vi "Test Panel Position.vi"() -> ()   [LabVIEW 2013]
uses:
  Type Defs/AD Settings.ctl
  Type Defs/Output Values.ctl
  Type Defs/Output Switches.ctl
  Type Defs/CO2 Settings.ctl
  Type Defs/Final Output for Dispaly 2.ctl
  Type Defs/Data Reading.ctl
  Type Defs/Named Final Output name list ordered.ctl
  Type Defs/All Timers.ctl
  Type Defs/Timer Control.ctl
  Altitude/Altitude.xctl
  Type Defs/Action Time.ctl
  Mode Control/Mode.xctl
  Type Defs/Current Alt Set.ctl
  Type Defs/Alt Control.ctl
  Type Defs/Alt Digit 100 New.ctl
  MSR/VertMode/VertMode.xctl
  Type Defs/Named Final Output name list with 02.ctl
  Type Defs/Alt Display Large.ctl
  <vilib>/Utility/miscctls.llb/LVPositionTypeDef.ctl
  <vilib>/Utility/miscctls.llb/LVRectTypeDef.ctl
  <vilib>/Utility/miscctls.llb/LVPointTypeDef.ctl
panel:
  out "Position":T1
  out "read string":string="Ver. 0.9, May 29 2013, 00:37:20\r\n"
  in  "Main Tabs":T2(tab)=enum."CO2 Settings"
  in  "Other Outputs":cluster{"Alarm":bool, "Heater":bool}
  out "CO2 ppm":u32(slide)=493 scale=0.0..10000.0
  out "Alt Dif":dbl(slide)=1604.2180978990014 scale=-1000.0..1000.0 scale format="%.1f"
  out "AD Output":T3
  out "AD State":T3
  out "Data Read":T4={"Date"="06/07/13", "Time"="14:45:26", "CO2- ppm"=493, "Last Ctrl Word"=12582912, "O2-1 ppm"=209797, "O2-2 ppm"=209799, "Temp MB"=26.17, "Temp Sensor Module"=27.17, "Press mB"=833.31} {"Last Ctrl Word" format="%.0x"}
  out "Force Output":T3
  out "Final Output":T3
  out "Force State":T3
  in  "CO2 Settings":T5={"Run C1"={"A-1,  1"=inf, "A-3,  2"=inf, "A-4, 3"=9600.0, "A-5, 4"=8800.0, "ABCD-7, 5"=9800.0, "A-8, 6"=9800.0, "B-1,  7"=3400.0, "B-3, 8"=3400.0, "B-4,  9"=9600.0, "B-5, 10"=8800.0, "B-8, 11"=9800.0, "C-1, 12"=1800.0, "C-3, 13"=1800.0, "C-4, 14"=9600.0, "C-5,  15"=8800.0, "C-8, 16"=9800.0, "D-1, 17"=inf, "D-3, 18"=3400.0, "D-4,  19"=1800.0, "D-5,  20"=9800.0, "D-8,  21"=9800.0}, "Run C2"={"A-1,  1"=inf, "A-3,  2"=inf, "A-4, 3"=9500.0, "A-5, 4"=8600.0, "ABCD-7, 5"=9700.0, "A-8, 6"=9700.0, "B-1,  7"=3000.0, "B-3, 8"=3000.0, "B-4,  9"=9500.0, "B-5, 10"=8600.0, "B-8, 11"=9700.0, "C-1, 12"=1400.0, "C-3, 13"=1400.0, "C-4, 14"=9500.0, "C-5,  15"=8600.0, "C-8, 16"=9700.0, "D-1, 17"=inf, "D-3, 18"=3000.0, "D-4,  19"=1400.0, "D-5,  20"=9700.0, "D-8,  21"=9700.0}, "Hold C3"={"A-1,  1"=1800.0, "A-3,  2"=1800.0, "A-4, 3"=9000.0, "A-5, 4"=8800.0, "ABCD-7, 5"=9800.0, "A-8, 6"=9800.0, "B-1,  7"=3400.0, "B-3, 8"=3400.0, "B-4,  9"=9000.0, "B-5, 10"=8800.0, "B-8, 11"=9800.0, "C-1, 12"=1800.0, "C-3, 13"=1800.0, "C-4, 14"=9000.0, "C-5,  15"=8800.0, "C-8, 16"=9800.0, "D-1, 17"=1800.0, "D-3, 18"=3400.0, "D-4,  19"=1800.0, "D-5,  20"=9800.0, "D-8,  21"=9800.0}, "Hold C4"={"A-1,  1"=1400.0, "A-3,  2"=1400.0, "A-4, 3"=8800.0, "A-5, 4"=8600.0, "ABCD-7, 5"=9700.0, "A-8, 6"=9700.0, "B-1,  7"=3000.0, "B-3, 8"=3000.0, "B-4,  9"=8800.0, "B-5, 10"=8600.0, "B-8, 11"=9700.0, "C-1, 12"=1400.0, "C-3, 13"=1400.0, "C-4, 14"=8800.0, "C-5,  15"=8600.0, "C-8, 16"=9700.0, "D-1, 17"=1400.0, "D-3, 18"=3000.0, "D-4,  19"=1400.0, "D-5,  20"=9700.0, "D-8,  21"=9700.0}, "High CO2 Forces"={"A-1, 1"=TRUE, "A-3, 2"=TRUE, "A-4, 3"=FALSE, "A-5, 4"=TRUE, "ABCD-7, 5"=FALSE, "A-8, 6"=TRUE, "B-1,  7"=TRUE, "B-3, 8"=TRUE, "B-4, 9"=FALSE, "B-5, 10"=TRUE, "B-8,  11"=TRUE, "C-1, 12"=TRUE, "C-3, 13"=TRUE, "C-4,  14"=FALSE, "C-5,  15"=TRUE, "C-8, 16"=TRUE, "D-1, 17"=TRUE, "D-3, 18"=TRUE, "D-4, 19"=TRUE, "D-5,  20"=TRUE, "D-8,  21"=TRUE}}
  in  "AD Settings":T8={"Set Point Force"={"A-1,  1"=inf, "A-3,  2"=inf, "A-4, 3"=inf, "A-5, 4"=5790.0, "ABCD-7, 5"=inf, "A-8, 6"=inf, "B-1,  7"=5790.0, "B-3, 8"=5790.0, "B-4,  9"=inf, "B-5, 10"=5790.0, "B-8, 11"=inf, "C-1, 12"=inf, "C-3, 13"=inf, "C-4, 14"=inf, "C-5,  15"=5790.0, "C-8, 16"=inf, "D-1, 17"=inf, "D-3, 18"=inf, "D-4,  19"=inf, "D-5,  20"=inf, "D-8,  21"=inf}, "Run A1"={"A-1,  1"=inf, "A-3,  2"=inf, "A-4, 3"=3.0, "A-5, 4"=inf, "ABCD-7, 5"=67.0, "A-8, 6"=630.0, "B-1,  7"=-30.0, "B-3, 8"=-30.0, "B-4,  9"=3.0, "B-5, 10"=inf, "B-8, 11"=630.0, "C-1, 12"=-60.0, "C-3, 13"=-60.0, "C-4, 14"=3.0, "C-5,  15"=inf, "C-8, 16"=630.0, "D-1, 17"=inf, "D-3, 18"=-30.0, "D-4,  19"=-60.0, "D-5,  20"=630.0, "D-8,  21"=930.0}, "Run A2"={"A-1,  1"=inf, "A-3,  2"=inf, "A-4, 3"=-3.0, "A-5, 4"=inf, "ABCD-7, 5"=60.0, "A-8, 6"=610.0, "B-1,  7"=-100.0, "B-3, 8"=-100.0, "B-4,  9"=-3.0, "B-5, 10"=inf, "B-8, 11"=610.0, "C-1, 12"=-120.0, "C-3, 13"=-120.0, "C-4, 14"=-3.0, "C-5,  15"=inf, "C-8, 16"=610.0, "D-1, 17"=inf, "D-3, 18"=-100.0, "D-4,  19"=-120.0, "D-5,  20"=610.0, "D-8,  21"=910.0}, "Hold A3"={"A-1,  1"=0.0, "A-3,  2"=0.0, "A-4, 3"=3.0, "A-5, 4"=inf, "ABCD-7, 5"=67.0, "A-8, 6"=630.0, "B-1,  7"=-150.0, "B-3, 8"=-150.0, "B-4,  9"=3.0, "B-5, 10"=inf, "B-8, 11"=630.0, "C-1, 12"=-300.0, "C-3, 13"=-300.0, "C-4, 14"=3.0, "C-5,  15"=inf, "C-8, 16"=630.0, "D-1, 17"=0.0, "D-3, 18"=-150.0, "D-4,  19"=-300.0, "D-5,  20"=630.0, "D-8,  21"=930.0}, "Hold A4"={"A-1,  1"=-150.0, "A-3,  2"=-150.0, "A-4, 3"=-3.0, "A-5, 4"=inf, "ABCD-7, 5"=60.0, "A-8, 6"=610.0, "B-1,  7"=-250.0, "B-3, 8"=-250.0, "B-4,  9"=-3.0, "B-5, 10"=inf, "B-8, 11"=610.0, "C-1, 12"=-500.0, "C-3, 13"=-500.0, "C-4, 14"=-3.0, "C-5,  15"=inf, "C-8, 16"=610.0, "D-1, 17"=-150.0, "D-3, 18"=-250.0, "D-4,  19"=-500.0, "D-5,  20"=610.0, "D-8,  21"=910.0}, "High AD Diff "={"A-1, 1"=FALSE, "A-3, 2"=FALSE, "A-4, 3"=FALSE, "A-5, 4"=TRUE, "ABCD-7, 5"=FALSE, "A-8, 6"=TRUE, "B-1,  7"=FALSE, "B-3, 8"=FALSE, "B-4, 9"=FALSE, "B-5, 10"=TRUE, "B-8,  11"=TRUE, "C-1, 12"=FALSE, "C-3, 13"=FALSE, "C-4,  14"=FALSE, "C-5,  15"=TRUE, "C-8, 16"=TRUE, "D-1, 17"=FALSE, "D-3, 18"=FALSE, "D-4, 19"=FALSE, "D-5,  20"=TRUE, "D-8,  21"=TRUE}, "Delay S"={"A-1,  1"=30.0, "A-3,  2"=30.0, "A-4, 3"=1.0, "A-5, 4"=1.0, "ABCD-7, 5"=1.0, "A-8, 6"=1.0, "B-1,  7"=30.0, "B-3, 8"=30.0, "B-4,  9"=1.0, "B-5, 10"=1.0, "B-8, 11"=1.0, "C-1, 12"=30.0, "C-3, 13"=30.0, "C-4, 14"=1.0, "C-5,  15"=1.0, "C-8, 16"=1.0, "D-1, 17"=30.0, "D-3, 18"=30.0, "D-4,  19"=30.0, "D-5,  20"=1.0, "D-8,  21"=1.0}}
  in  "Main States":T9(tab)
  out "ALT DISPLAY":dbl format="%#.0f"
  out "Heading":string="Current Effective Altitude in  Feet"
  out "CURRENT ALT SET":T10 caption="Current Set Point" format="%#.0f"
  in  "Mode 1":enum8{"Off", "Stby", "Hold", "Run"}(xcontrol)=enum."Stby"
  in  "Confirm Now 2":bool
  out "Carbon Dioxide  %":sgl format="%.3f"
  in  "ALT SET 2":T11 {"Alt Digit 100" min=0 max=9 step=1; "Alt Digit 100" min=0 max=9 step=1; "Alt Digit 100" min=0 max=9 step=1; "Alt Digit 100" min=0 max=9 step=1; "Alt Digit 100" min=0 max=9 step=1}
  out "ALT DISPLAY 2":T13 format="%#.0f"
  out "Comm Error 2":bool caption="Sensor Connection"
  out "Heading 2":string="Current Effective Altitude in  Feet"
  out "CURRENT ALT SET 2":T10 caption="Current Set Point" format="%#.0f"
  out "Time":string="14:45:20"
  in  "Add Note":bool
  out "CO2 Chart":sgl(graph)
  out "Temp C":sgl=26.28
  out "Press mB":sgl=833.25
  out "Date":string="06/07/13"
  out "Alt Chart":sgl(graph)
  out "Carbon Dioxide %":sgl=0.0493 format="%.3g"
  in  "Confirm Now":bool
  in  "Notes":string
  in  "ALT SET":T11 {"Alt Digit 100" min=0 max=9 step=1; "Alt Digit 100" min=0 max=9 step=1; "Alt Digit 100" min=0 max=9 step=1; "Alt Digit 100" min=0 max=9 step=1; "Alt Digit 100" min=0 max=9 step=1}
  out "Altitude":sgl format="%#.0f"
  out "O2%":sgl=20.9793 format="%.2f"
  out "Comm Error":bool caption="Connection"
  out "Numeric":i32=66
  out "Units":string="F\ne\ne\nt"
  in  "Mode":enum8{"Off", "Stby", "Hold", "Run"}(xcontrol)=enum."Stby"
  out "Final  Output Names":T14={"A-1,  1"="Main", "A-3,  2"="Main", "A-4, 3"="Recircirculation", "A-5, 4"="Scrubber", "A-7, 5"="Oxygen", "A-8, 6"="Vent", "B-1,  7"="Boost A", "B-3, 8"="Boost A", "B-4,  9"="Recircirculation", "B-5, 10"="Scrubber", "B-8, 11"="Vent", "C-1, 12"="Boost B", "C-3, 13"="Boost B", "C-4, 14"="Recircirculation", "C-5,  15"="Scrubber", "C-8, 16"="Vent", "D-1, 17"="Main", "D-3, 18"="Boost A", "D-4,  19"="Boost B", "D-5,  20"="Vent", "D-8,  21"="Vent 2", "B-7"="Oxygen", "C-7"="Oxygen", "D-7"="Oxygen", "A-1"=FALSE, "A-3"=FALSE, "A-4"=FALSE, "A-5"=FALSE, "A-7"=FALSE, "A-8"=FALSE, "B-1"=FALSE, "B-3"=FALSE, "B-4"=FALSE, "B-5"=FALSE, "B-7"=FALSE, "B-8"=FALSE, "C-1"=FALSE, "C-3"=FALSE, "C-4"=FALSE, "C-5"=FALSE, "C-7"=FALSE, "C-8"=FALSE, "D-1"=FALSE, "D-3"=FALSE, "D-4"=FALSE, "D-5"=FALSE, "D-7"=FALSE, "D-8"=FALSE}
  in  "Timers":T15 {"Timer 4"."Action Time" format="%<%H:%M>t"; "Timer 3"."Action Time" format="%<%H:%M>t"; "Timer 2"."Action Time" format="%<%H:%M>t"; "Timer"."Action Time" format="%<%H:%M>t"}
  out "Setup Tab":T18(tab)
  out "System Locked, Contact CAT":bool
  out "Days Until Factory Service":u32
  out "Days Until Calibration":u32
  out "Days Since Calibration":u32
  in  "Datalog File":path
  in  "Room or Project Name":string
  in  "Feet OFF/ Meters ON":bool
  in  "ALT Window ON/OFF":bool
  in  "PBaro":bool
  in  "Timers ON/OFF":bool
  out "Current PBaro":dbl
  in  "PBaro Fixed":dbl
  in  "Enter Calibration":bool
  in  "Screen 2 Password":string
  in  "Screen 1 Password":string
  in  "West ON/Std OFF":bool
  in  "maxAltSP":sgl caption="Maximum Altitude Setpoint"
  in  "Save Names":bool
  in  "Load Names":bool
  in  "Setup Tables Visible":bool
  in  "Period mS":i64=6000
  in  "Final  Output Names  2":T19={"A-1, 1"="Main", "A-3, 2"="Main", "A-4, 3"="Recircirculation", "A-5, 4"="Scrubber", "A-7, 5"="Oxygen", "A-8, 6"="Vent", "B-1,  7"="Boost A", "B-3, 8"="Boost A", "B-4, 9"="Recircirculation", "B-5, 10"="Scrubber", "B-8, 11"="Vent", "C-1, 12"="Boost B", "C-3, 13"="Boost B", "C-4, 14"="Recircirculation", "C-5,  15"="Scrubber", "C-8, 16"="Vent", "D-1, 17"="Main", "D-3, 18"="Boost A", "D-4,  19"="Boost B", "D-5,  20"="Vent", "D-8,  21"="Vent 2"}
  in  "Enter or Exit Setup":bool
  in  "Stop Button":bool=TRUE
  out "Error Report Status":errorcluster
  out "Cycles":i32=10
  in  "Set Point Alt":sgl min=0 max=10000 step=1
  # "CAT 100.98"
  # "Channel A"
  # "Channel B"
  # "Channel C"
  # "Channel D"
  # "Channel A"
  # "Channel B"
  # "Channel C"
  # "Channel D"
  # "Channel A"
  # "Channel B"
  # "Channel C"
  # "Channel D"
  # "Channel A"
  # "Channel B"
  # "Channel C"
  # "Channel D"
  # "Channel A"
  # "Channel B"
  # "Channel C"
  # "Channel D"
  # "Channel A"
  # "Channel B"
  # "Channel C"
  # "Channel D"
  # "1"
  # "1"
  # "1"
  # "1"
  # "Altiude Adjustment Controls"
  # "Time and Date Set Here"
types:
  T1 = typedef "LVPositionTypeDef.ctl" = cluster{"Left":i32, "Top":i32}
  T2 = enum32{"Inputs and Controls", "CO2 and AD Outputs", "CO2 Settings", "AD Settings"}
  T3 = typedef "Final Output for Dispaly 2.ctl" = cluster{"A-1,  1":bool, "A-3,  2":bool, "A-4, 3":bool, "A-5, 4":bool, "ABCD-7, 5":bool, "A-8, 6":bool, "B-1,  7":bool, "B-3, 8":bool, "B-4,  9":bool, "B-5, 10":bool, "B-8, 11":bool, "C-1, 12":bool, "C-3, 13":bool, "C-4, 14":bool, "C-5,  15":bool, "C-8, 16":bool, "D-1, 17":bool, "D-3, 18":bool, "D-4,  19":bool, "D-5,  20":bool, "D-8,  21":bool}
  T4 = typedef "Data Reading.ctl" = cluster{"Date":string, "Time":string, "CO2- ppm":u32, "Last Ctrl Word":u32, "O2-1 ppm":u32, "O2-2 ppm":u32, "Temp MB":sgl, "Temp Sensor Module":sgl, "Press mB":sgl}
  T5 = typedef "CO2 Settings.ctl" = cluster{"Run C1":T6, "Run C2":T6, "Hold C3":T6, "Hold C4":T6, "High CO2 Forces":T7}
  T6 = typedef "Output Values.ctl" = cluster{"A-1,  1":dbl, "A-3,  2":dbl, "A-4, 3":dbl, "A-5, 4":dbl, "ABCD-7, 5":dbl, "A-8, 6":dbl, "B-1,  7":dbl, "B-3, 8":dbl, "B-4,  9":dbl, "B-5, 10":dbl, "B-8, 11":dbl, "C-1, 12":dbl, "C-3, 13":dbl, "C-4, 14":dbl, "C-5,  15":dbl, "C-8, 16":dbl, "D-1, 17":dbl, "D-3, 18":dbl, "D-4,  19":dbl, "D-5,  20":dbl, "D-8,  21":dbl}
  T7 = typedef "Output Switches.ctl" = cluster{"A-1, 1":bool, "A-3, 2":bool, "A-4, 3":bool, "A-5, 4":bool, "ABCD-7, 5":bool, "A-8, 6":bool, "B-1,  7":bool, "B-3, 8":bool, "B-4, 9":bool, "B-5, 10":bool, "B-8,  11":bool, "C-1, 12":bool, "C-3, 13":bool, "C-4,  14":bool, "C-5,  15":bool, "C-8, 16":bool, "D-1, 17":bool, "D-3, 18":bool, "D-4, 19":bool, "D-5,  20":bool, "D-8,  21":bool}
  T8 = typedef "AD Settings.ctl" = cluster{"Set Point Force":T6, "Run A1":T6, "Run A2":T6, "Hold A3":T6, "Hold A4":T6, "High AD Diff ":T7, "Delay S":T6}
  T9 = enum32{"Altitude", "Simple Display", "Detailed Display", "Timers", "Setup"}
  T10 = typedef "Current Alt Set.ctl" = i32
  T11 = typedef "Alt Control.ctl" = cluster{"Alt Digit 100":T12, "Alt Digit 100":T12, "Alt Digit 100":T12, "Alt Digit 100":T12, "Alt Digit 100":T12}
  T12 = typedef "Alt Digit 100 New.ctl" = i8
  T13 = typedef "Alt Display Large.ctl" = sgl
  T14 = typedef "Named Final Output name list with 02.ctl" = cluster{"A-1,  1":string, "A-3,  2":string, "A-4, 3":string, "A-5, 4":string, "A-7, 5":string, "A-8, 6":string, "B-1,  7":string, "B-3, 8":string, "B-4,  9":string, "B-5, 10":string, "B-8, 11":string, "C-1, 12":string, "C-3, 13":string, "C-4, 14":string, "C-5,  15":string, "C-8, 16":string, "D-1, 17":string, "D-3, 18":string, "D-4,  19":string, "D-5,  20":string, "D-8,  21":string, "B-7":string, "C-7":string, "D-7":string, "A-1":bool, "A-3":bool, "A-4":bool, "A-5":bool, "A-7":bool, "A-8":bool, "B-1":bool, "B-3":bool, "B-4":bool, "B-5":bool, "B-7":bool, "B-8":bool, "C-1":bool, "C-3":bool, "C-4":bool, "C-5":bool, "C-7":bool, "C-8":bool, "D-1":bool, "D-3":bool, "D-4":bool, "D-5":bool, "D-7":bool, "D-8":bool}
  T15 = typedef "All Timers.ctl" = cluster{"Timer":T16, "Timer 2":T16, "Timer 3":T16, "Timer 4":T16}
  T16 = typedef "Timer Control.ctl" = cluster{"Sun":bool, "Timer":bool, "Altitude":sgl, "Action Time":T17, "Mon":bool, "Tues":bool, "Wed":bool, "Thur":bool, "Fri":bool, "Sat":bool, "Mode":enum8{"Off", "Stby", "Hold", "Run"}}
  T17 = typedef "Action Time.ctl" = dbl
  T18 = enum32{"Setup 0", "Setup 1", "Setup 2", "Setup 3"}
  T19 = typedef "Named Final Output name list ordered.ctl" = cluster{"A-1, 1":string, "A-3, 2":string, "A-4, 3":string, "A-5, 4":string, "A-7, 5":string, "A-8, 6":string, "B-1,  7":string, "B-3, 8":string, "B-4, 9":string, "B-5, 10":string, "B-8, 11":string, "C-1, 12":string, "C-3, 13":string, "C-4, 14":string, "C-5,  15":string, "C-8, 16":string, "D-1, 17":string, "D-3, 18":string, "D-4,  19":string, "D-5,  20":string, "D-8,  21":string}
  T20 = typedef "LVPointTypeDef.ctl" = cluster{"Horizontal":i16, "Vertical":i16}
  T21 = enum16{"Always On", "Always Off", "Off While Running"}
  T22 = typedef "LVRectTypeDef.ctl" = cluster{"Left":i16, "Top":i16, "Right":i16, "Bottom":i16}
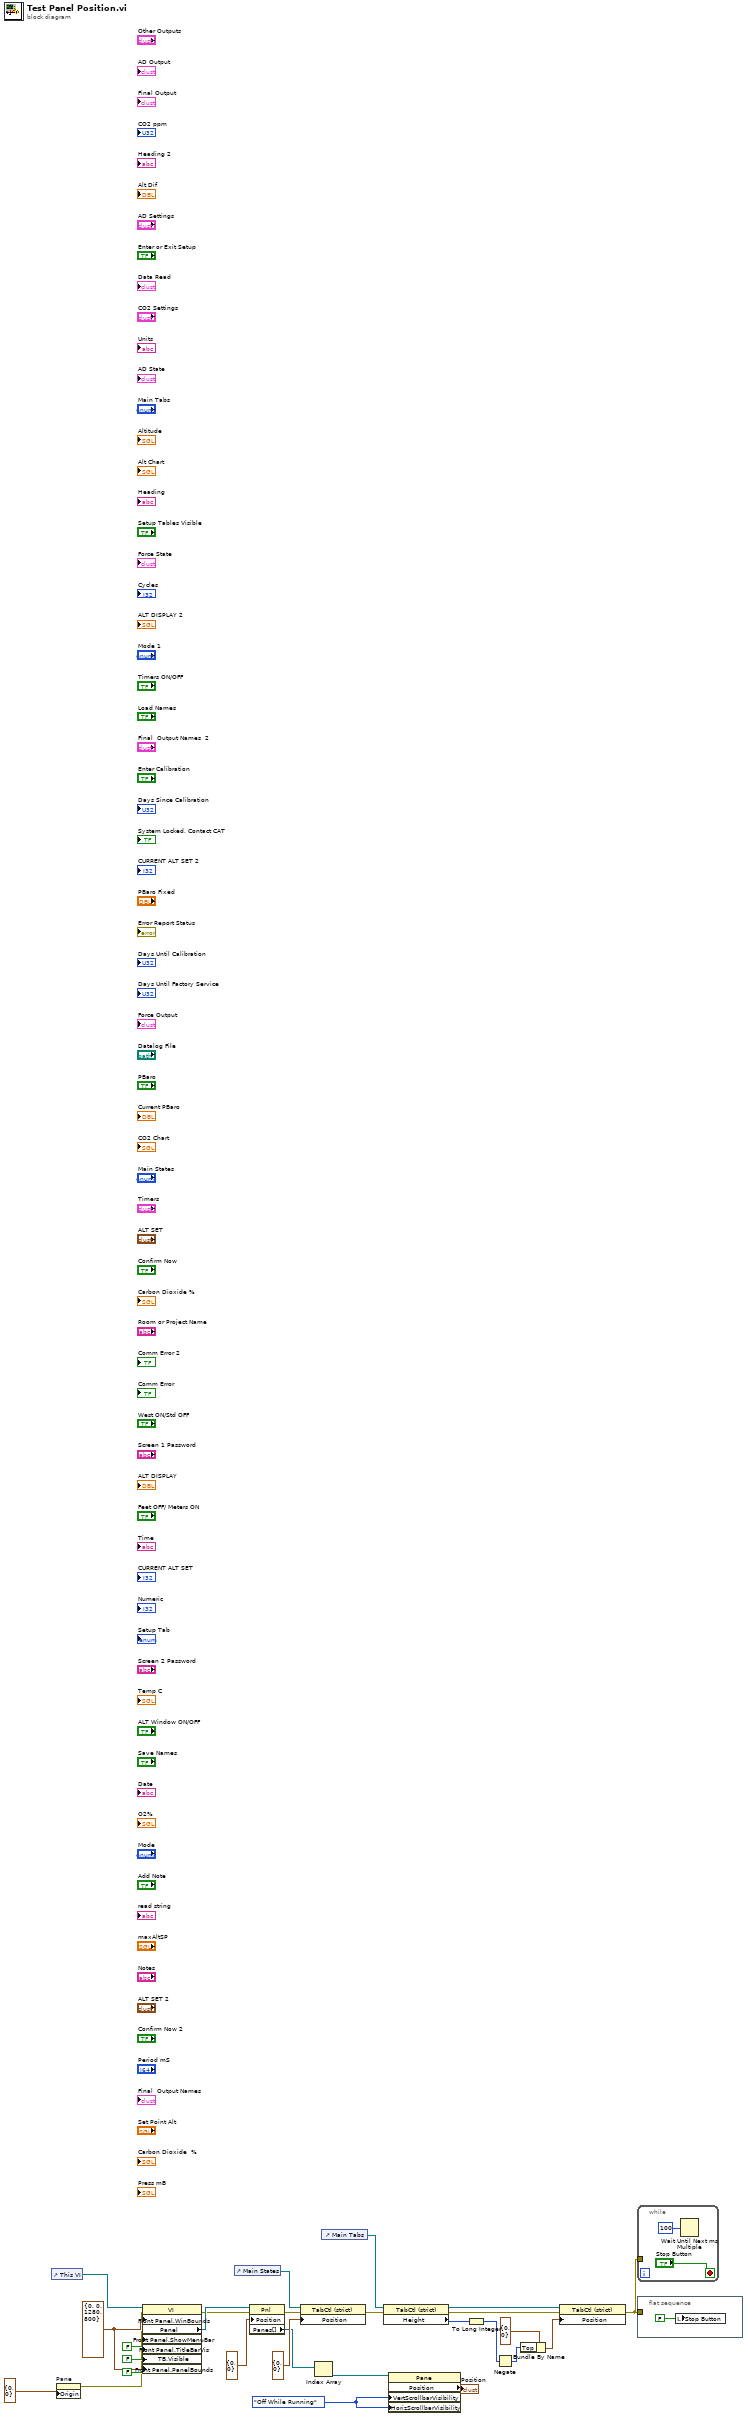
[diagram p0: block diagram]
diagram:
  w3 = T21."Off While Running" ("Vertical Scrollbar Visibility")
  w4 = T22 {"Left"=0, "Top"=0, "Right"=1280, "Bottom"=800} ("Front Panel Window:Window Bounds")
  n1 = control-ref of="This VI"() -> (w27:refnum<vi>)
  n2 = property on="Pane" class="Pane"("Origin"=T20 {"Horizontal"=0, "Vertical"=0}) -> (error out=w1:errorcluster)  [unwired: 2 in, 1 out]
  n3 = property class="VI"(reference=w27, error in=w1, "Front Panel.WinBounds"=w4, "Front Panel.ShowMenuBar"=FALSE ("Front Panel Window:Show Menu Bar"), "Front Panel.TitleBarVis"=FALSE ("Front Panel Window:Title Bar Visible"), "TB.Visible"=FALSE ("Tool Bar:Visible"), "Front Panel.PanelBounds"=w4) -> (error out=w22:errorcluster, "Panel"=w24:refnum<vi>)  [unwired: 1 out]
  n4 = control-ref of="Main States"() -> (w26:refnum<vi>)
  n5 = property class="Pnl"(reference=w24, error in=w22, "Position"=T1 {"Left"=0, "Top"=0}) -> (error out=w21:errorcluster, "Panes[]"=w10:refnum<vi>[])  [unwired: 1 out]
  n6 = property class="TabCtl (strict)"(reference=w26, error in=w21, "Position"=T1 {"Left"=0, "Top"=0}) -> (error out=w13:errorcluster)  [unwired: 1 out]
  n7 = Index Array(array=w10) -> (element=w9:refnum<vi>)  [unwired: 1 in]
  n8 = control-ref of="Main Tabs"() -> (w20:refnum<vi>)
  n9 = property class="TabCtl (strict)"(reference=w20, error in=w13) -> (reference out=w19:refnum<vi>, error out=w12:errorcluster, "Height"=w17:u32)
  n10 = property class="Pane"(reference=w9, "VertScrollbarVisibility"=w3, "HorizScrollbarVisibility"=w3) -> ("Position"=→"Position":T1)  [unwired: 1 in, 2 out]
  n11 = To Long Integer(number=w17) -> (32bit integer=w18:i32)
  n12 = Negate(x=w18) -> (-x=w15:i32)
  n13 = Bundle By Name(cluster=T1 {"Left"=0, "Top"=0} ("Position"), "Top"=w15) -> (w14:T1)
  n14 = property class="TabCtl (strict)"(reference=w19, error in=w12, "Position"=w14) -> (error out=w11:errorcluster)  [unwired: 1 out]
  n15 = while {
    tunnel: w11 -> [_]
    stop <- "Stop Button" stop-if-true
    n16 = Wait Until Next ms Multiple(millisecond multiple=u32 100) -> ()  [unwired: 1 out]
  }
  n17 = flat-sequence {
    tunnel: w11 -> [_]
    frame #0 {
      n18 = local write "Stop Button"(FALSE ("Stop Button")) -> ()
    }
  }
